vi "ProducerConsumerEvents_Events_Medicao.vi"() -> ()   [LabVIEW 2026]
doc: "Use this template to build a producer/consumer design pattern with events to produce queue items. Use this design pattern instead of the User Interface Event Handler pattern for user interfaces when you want to execute code asynchronously in response to an event without slowing the user interface responsiveness."
uses:
  <vilib>/Instr/_visa.llb/VISA Configure Serial Port (Instr).vi
panel:
  in  "Read":bool
  in  "Dial":dbl(knob) scale=0.0..3.3
  out "Status Motor":bool
  in  "stop 3":bool
  in  "?":bool
  in  "Write":bool
  in  "stop 2":bool
  out "Humidity":dbl(graph)
  out "Temperature":dbl(graph)
  in  "stop":bool
  out "read buffer":string
  out "error out":errorcluster
  in  "Read Count":u32=1000
  out "Response":string
  in  "Termination Character":u8=10 format="%.0x"
  in  "VISA resource name":refnum<visa-resource-name>="COM1"
  in  "Serial Settings":T1={"baud rate"=9600, "data bits"=8, "parity"=enum."None", "stop bits"=10, "flow control"=0} {"flow control" items=["None"=0, "XON/XOFF"=1, "RTS/CTS"=2, "DTR/DSR"=4]; "stop bits" items=["1.0"=10, "1.5"=15, "2.0"=20]; "data bits" min=5 max=8 step=1; "baud rate" items=["75"=75, "110"=110, "134"=134, "150"=150, "300"=300, "600"=600, "1200"=1200, "1800"=1800, "2400"=2400, "4800"=4800, "7200"=7200, "9600"=9600, "14400"=14400, "19200"=19200, "28800"=28800, "38400"=38400, "56000"=56000, "57600"=57600, "115200"=115200, "128000"=128000, "230400"=230400]}
  in  "End Read on Termination Character?":bool=TRUE
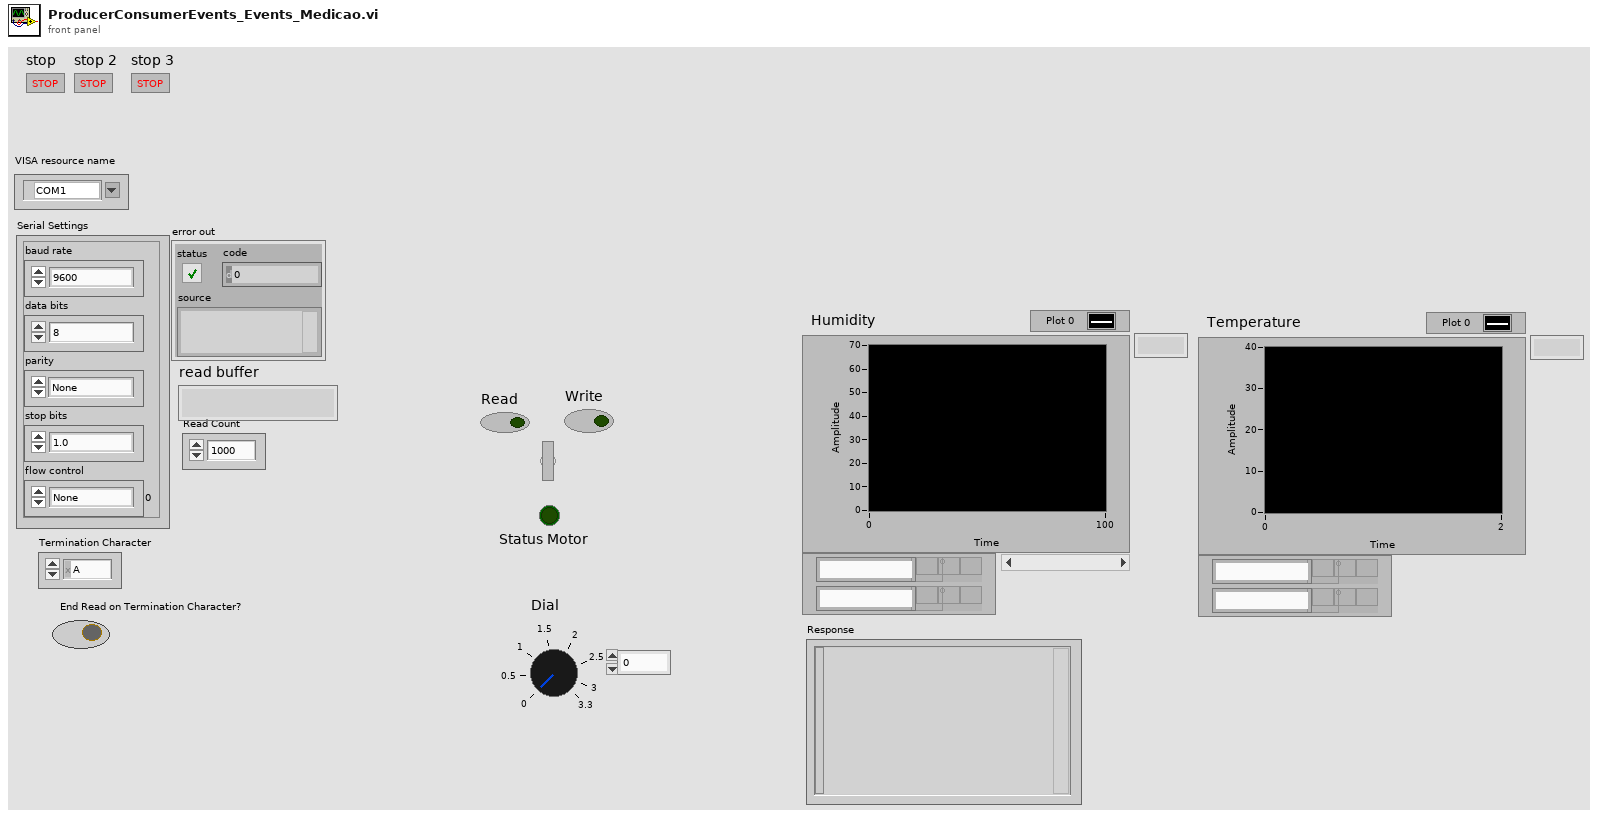
[diagram p1: front panel]
types:
  T1 = cluster{"baud rate":u32, "data bits":u16, "parity":enum16{"None", "Odd", "Even", "Mark", "Space"}, "stop bits":u16, "flow control":u16}
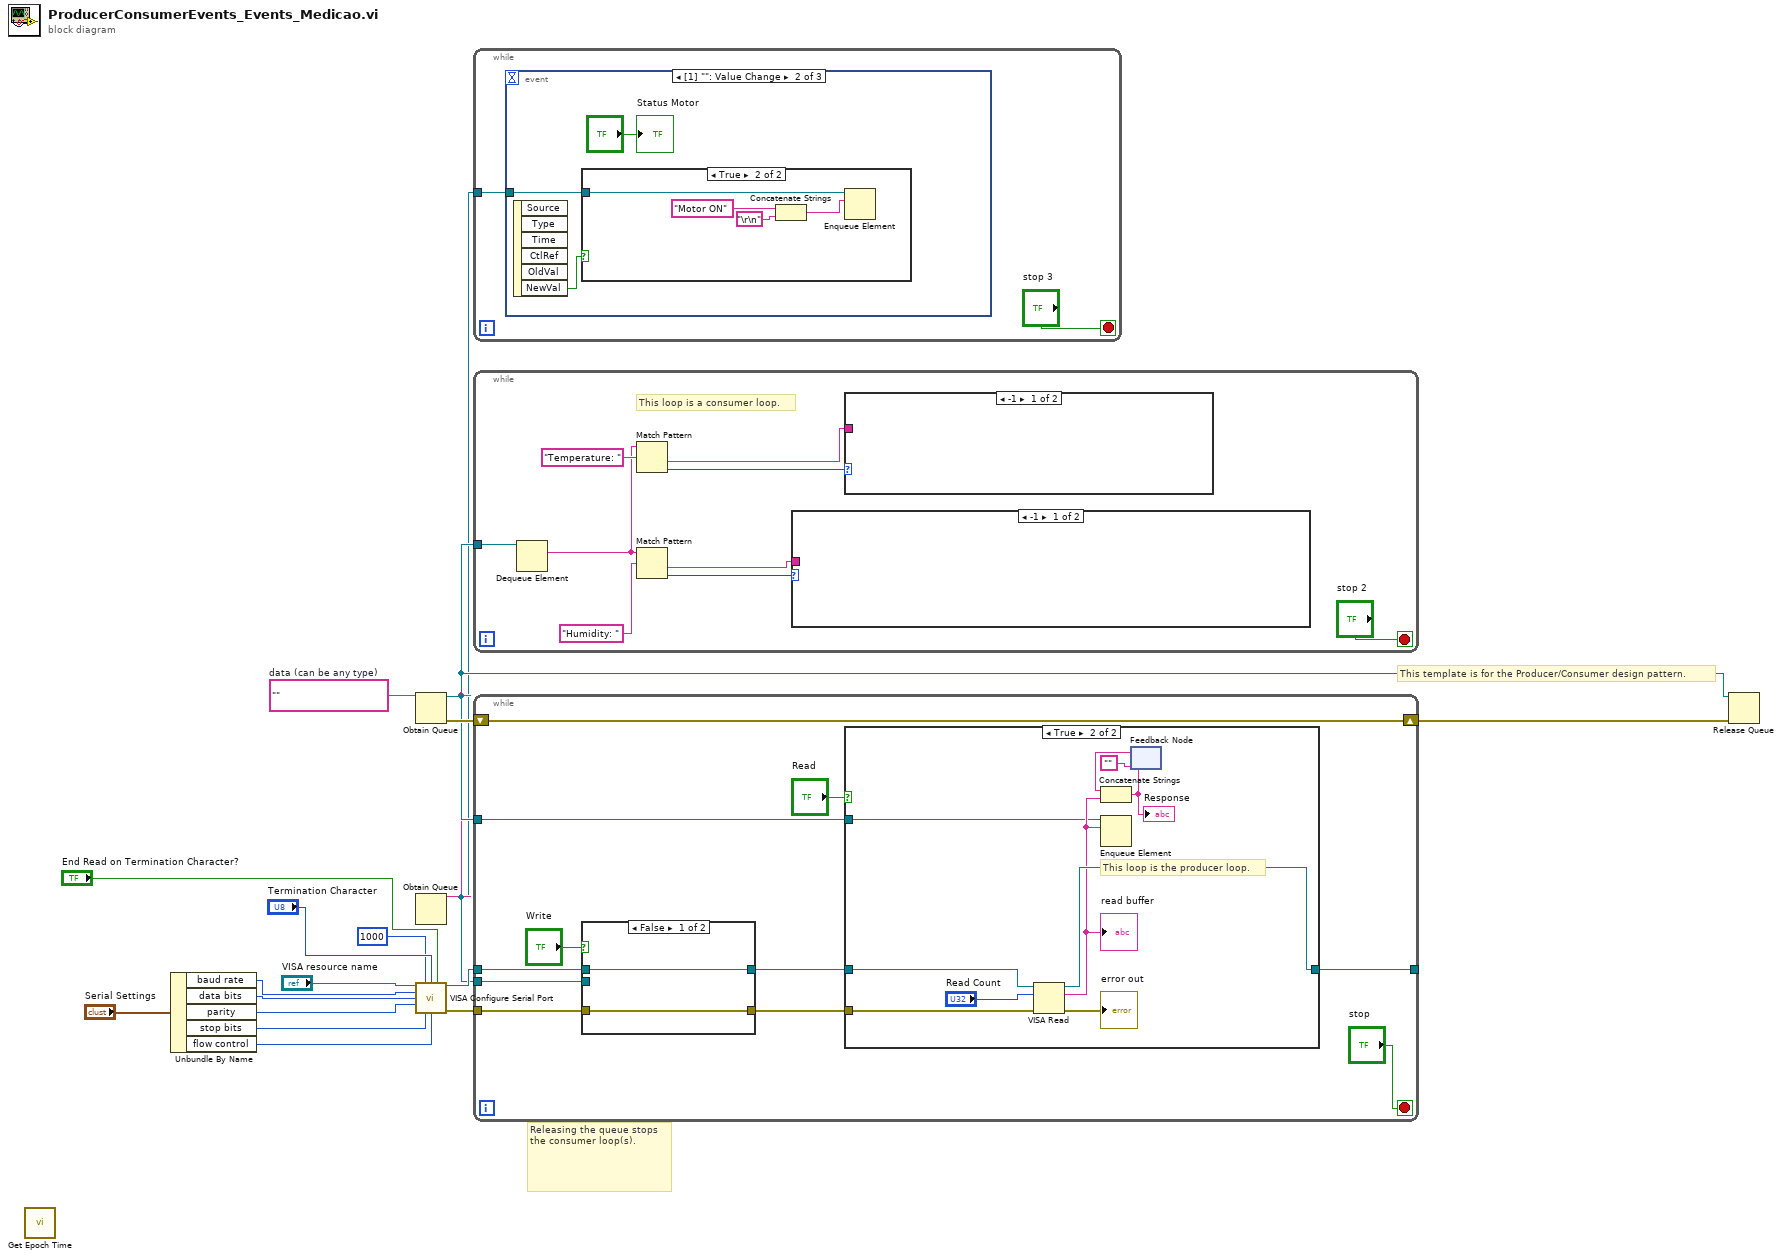
[diagram p0: block diagram]
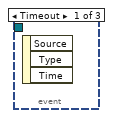
[diagram p2: hidden frame]
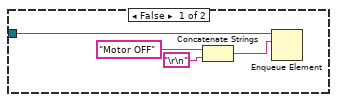
[diagram p3: hidden frame]
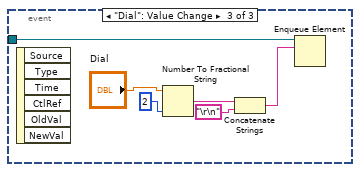
[diagram p4: hidden frame]
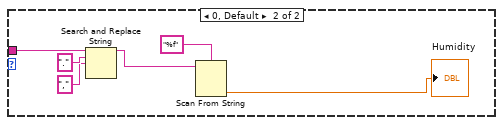
[diagram p5: hidden frame]
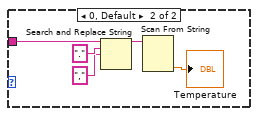
[diagram p6: hidden frame]
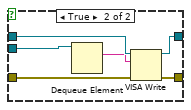
[diagram p8: hidden frame]
diagram:
  w3 = ""  # data (can be any type)
  # "Releasing the queue stops the consumer loop(s)."
  # "This template is for the Producer/Consumer design pattern."
  n1 = call <vilib>:"Get Epoch Time.vi"() -> ()  [unwired: 9 in, 3 out]
  n2 = Unbundle By Name("Serial Settings") -> ("baud rate"=w10:u32, "data bits"=w9:u16, "parity"=w8:enum16{"None", "Odd", "Even", "Mark", "Space"}, "stop bits"=w7:u16, "flow control"=w13:u16)
  n3 = Obtain Queue(element data type=w3) -> (queue out=w15:refnum<queue>, error out=w17:errorcluster)  [unwired: 4 in, 1 out]
  n4 = Obtain Queue(element data type=w3) -> (queue out=w2:refnum<queue>)  [unwired: 4 in, 2 out]
  n5 = call-poly "VISA Configure Serial Port"("VISA resource name"="VISA resource name", "timeout (10sec)"=u32 1000, "termination char\n(0xA = '\\n' = LF)"="Termination Character", "Enable Termination\nChar (T)"="End Read on Termination Character?", "baud rate (9600)"=w10, "data bits (8)"=w9, "parity (0:none)"=w8, "stop bits (10: 1 bit)"=w7, "flow control (0:none)"=w13) -> ("VISA resource name out"=w5:refnum<visa-resource-name>, "error out"=w4:errorcluster)  [unwired: 1 in, 4 out]
  n6 = while {
    tunnel: w2 -> [w18]
    stop <- "stop 3" stop-if-true
    n7 = event shown="[1] \"\": Value Change" {
      selector: _ -> [_ _ _]
      dyn-events: _ -> [_ _ _]
      timeout: _ -> [_ _ _]
      tunnel: w18 -> [_ w22 w36]
      event Timeout {
        n8 = event-data() -> ()  [unwired: 1 in, 3 out]
      }
      event Value Change {
        n9 = event-data() -> ("NewVal"=w21:bool)  [unwired: 1 in, 5 out]
        n10 = case shown="True" w21 {
          tunnel: w22 -> [w26 w30]
          frame False {
            n11 = Concatenate Strings("Motor OFF", "\r\n") -> (w24:string)
            n12 = Enqueue Element(queue=w26, element=w24) -> ()  [unwired: 2 in, 3 out]
          }
          frame True {
            n13 = Concatenate Strings("Motor ON", "\r\n") -> (w27:string)
            n14 = Enqueue Element(queue=w30, element=w27) -> ()  [unwired: 2 in, 3 out]
          }
        }
        "Status Motor" <- "?"
      }
      event "Dial": Value Change {
        n15 = event-data() -> ()  [unwired: 1 in, 6 out]
        n16 = Number To Fractional String(number="Dial", precision (6)=i16 2) -> (F-format string=w33:string)  [unwired: 2 in]
        n17 = Concatenate Strings(w33, "\r\n") -> (w31:string)
        n18 = Enqueue Element(queue=w36, element=w31) -> ()  [unwired: 2 in, 3 out]
      }
    }
  }
  n19 = while {
    tunnel: w15 -> [w45]
    stop <- "stop 2" stop-if-true
    # "This loop is a consumer loop."
    n20 = Dequeue Element(queue=w45) -> (element=w39:string)  [unwired: 2 in, 3 out]
    n21 = Match Pattern(string=w39, regular expression="Temperature: ") -> (after substring=w37:string, offset past match=w41:i32)  [unwired: 1 in, 2 out]
    n22 = Match Pattern(string=w39, regular expression="Humidity: ") -> (after substring=w42:string, offset past match=w40:i32)  [unwired: 1 in, 2 out]
    n23 = case shown="-1" w40 {
      tunnel: w42 -> [_ w49]
      frame -1 {
      }
      frame 0, Default {
        n24 = Search and Replace String(input string=w49, search string=".", replace string="," ("replace string (\"\")")) -> (result string=w46:string)  [unwired: 5 in, 3 out]
        n25 = Scan From String "Scan From String"(format string="%f", input string=w46) -> (output 1=→"Humidity":dbl)  [unwired: 3 in, 3 out]
      }
    }
    n26 = case shown="-1" w41 {
      tunnel: w37 -> [_ w55]
      frame -1 {
      }
      frame 0, Default {
        n27 = Search and Replace String(input string=w55, search string=".", replace string="," ("replace string (\"\")")) -> (result string=w54:string)  [unwired: 5 in, 3 out]
        n28 = Scan From String(input string=w54) -> (output 1=→"Temperature":dbl)  [unwired: 4 in, 3 out]
      }
    }
  }
  n29 = while {
    shift-right: [w64] -> w16
    shift-left: w17 -> [w64]
    tunnel: w15 -> [w66]
    tunnel: [w67] -> _
    tunnel: w5 -> [w63]
    tunnel: w4 -> [w62]
    tunnel: w2 -> [w58]
    stop <- "stop" stop-if-true
    n30 = case shown="False" "Write" {
      tunnel: w63 -> [w80 w86]
      tunnel: w62 -> [w79 w85]
      tunnel: [w80 w84] -> w59
      tunnel: [w79 w83] -> w61
      tunnel: w58 -> [_ w82]
      frame False {
      }
      frame True {
        n31 = Dequeue Element(queue=w82) -> (element=w81:string)  [unwired: 2 in, 3 out]
        n32 = VISA Write(VISA resource name=w86, write buffer=w81, error in (no error)=w85) -> (VISA resource name out=w84:refnum<visa-resource-name>, error out=w83:errorcluster)  [unwired: 1 out]
      }
    }
    n33 = case shown="True" "Read" {
      tunnel: [w68 w74] -> w67
      tunnel: w66 -> [_ w71]
      tunnel: w61 -> [_ w70]
      tunnel: w59 -> [w68 w69]
      frame False {
      }
      frame True {
        # "This loop is the producer loop."
        n34 = VISA Read(VISA resource name=w69, byte count="Read Count", error in (no error)=w70) -> (VISA resource name out=w74:refnum<visa-resource-name>, read buffer=w72:string, error out=→"error out":errorcluster)  [unwired: 1 out]
        "read buffer" <- w72
        n35 = Enqueue Element(queue=w71, element=w72) -> ()  [unwired: 2 in, 3 out]
        n36 = feedback #1("") -> (w77:string)
        n37 = Concatenate Strings(w77, w72) -> (w76:string)
        "Response" <- w76
        n38 = feedback-in #1(w76) -> ()
      }
    }
  }
  n39 = Release Queue(queue=w15, error in (no error)=w16) -> ()  [unwired: 1 in, 3 out]
